vi "Get Event-Timer.vi"(8 "error in (no error)":errorcluster, 11 "PDO Communication Parameter in":refnum<class "PDO Communication Parameter.lvclass">) -> (0 "error out":errorcluster, 2 "Event-Timer":u16, 3 "PDO Communication Parameter out":refnum<class "PDO Communication Parameter.lvclass">)   [LabVIEW 2020, in "CANopen.lvlib" / "PDO Communication Parameter.lvclass"]
uses:
  PDO Communication Parameter.lvclass
  PDO Communication Parameter.lvclass/PDO Communication Parameter.ctl
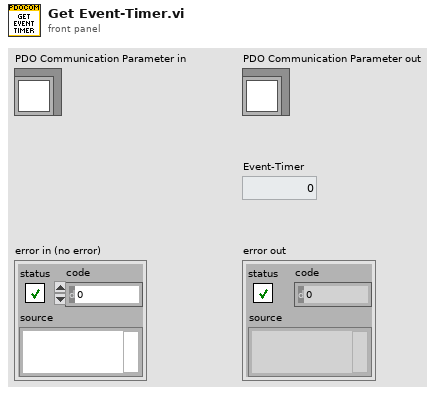
[diagram p1: front panel]
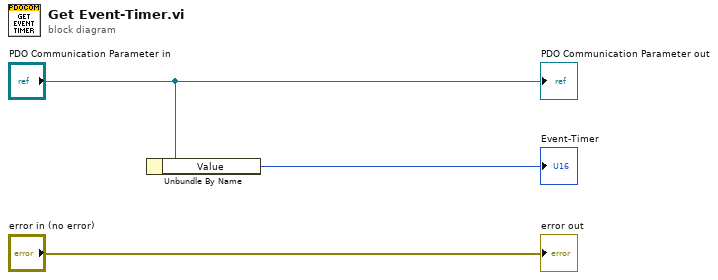
[diagram p0: block diagram]
diagram:
  n1 = Unbundle By Name("PDO Communication Parameter in") -> ("Value"=→"Event-Timer":u16)
  "error out" <- "error in (no error)"
  "PDO Communication Parameter out" <- "PDO Communication Parameter in"
